vi "Call About Dialog.vi"(8 "error in (no error)":errorcluster, 10 "AppVer":string, 11 "Main UI Ref":refnum<vi>) -> (0 "error out":errorcluster)   [LabVIEW 2019]
doc: "Developed by Kevin Thompson\nkevin@thompsonengineering.net\n\nCopyright 2018-2020\nThompson Engineering, LLC"
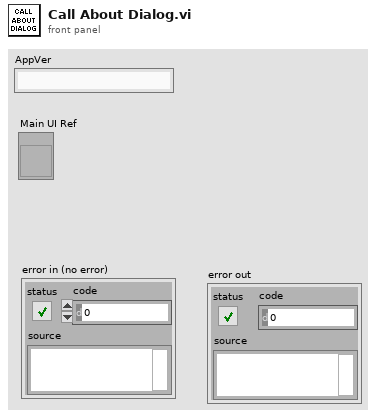
[diagram p1: front panel]
types:
  T1 = enum32{"Bad", "Idle", "Run top level", "Running"}
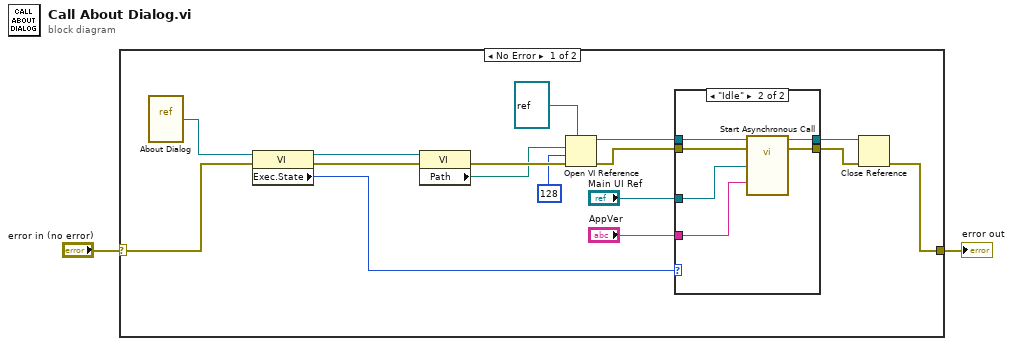
[diagram p0: block diagram]
diagram:
  n1 = case shown="No Error" "error in (no error)" {
    selector: "error in (no error)" -> [w7 w27]
    tunnel: [w14 w27] -> w2
    frame No Error {
      n2 = vi-ref "About Dialog.vi"() -> (w4:refnum<vi>)
      n3 = property class="VI"(reference=w4, error in=w7) -> (reference out=w9:refnum<vi>, error out=w12:errorcluster, "Exec.State"=w6:T1)
      n4 = property class="VI"(reference=w9, error in=w12) -> (error out=w13:errorcluster, "Path"=w10:path)  [unwired: 1 out]
      n5 = Open VI Reference(type specifier VI Refnum (for type only)=refnum<vi> refnum, vi path=w10, options=128, error in (no error)=w13) -> (vi reference=w8:refnum<vi>, error out=w5:errorcluster)  [unwired: 2 in]
      n6 = case shown="\"Idle\"" w6 {
        tunnel: "AppVer" -> [_ w26]
        tunnel: "Main UI Ref" -> [_ w25]
        tunnel: [w20 w24] -> w16
        tunnel: [w19 w23] -> w15
        tunnel: w8 -> [w20 w22]
        tunnel: w5 -> [w19 w21]
        frame "Bad", Default {
        }
        frame "Idle" {
          n7 = call-by-ref "Start Asynchronous Call"(reference=w22, error in=w21, "AppVer"=w26, "Main UI Ref"=w25) -> (reference out=w24:refnum<vi>, error out=w23:errorcluster)  [unwired: 2 in]
        }
      }
      n8 = Close Reference(reference=w16, error in (no error)=w15) -> (error out=w14:errorcluster)
    }
    frame Error {
    }
  }
  "error out" <- w2
